vi "Bool Array To Grid.vi"(8 "error in (no error)":errorcluster, 10 "Bool Array In":bool[](array[boolean]), 11 "ElectrodeGrid in":refnum<class "ElectrodeGrid.lvclass">) -> (0 "error out":errorcluster, 2 "Elec Grid Output":bool[][](array[boolean]), 3 "ElectrodeGrid out":refnum<class "ElectrodeGrid.lvclass">)   [LabVIEW 2017, in "ElectrodeGrid.lvclass"]
uses:
  ElectrodeGrid.lvclass
  ElectrodeGrid.lvclass/ElectrodeGrid.ctl
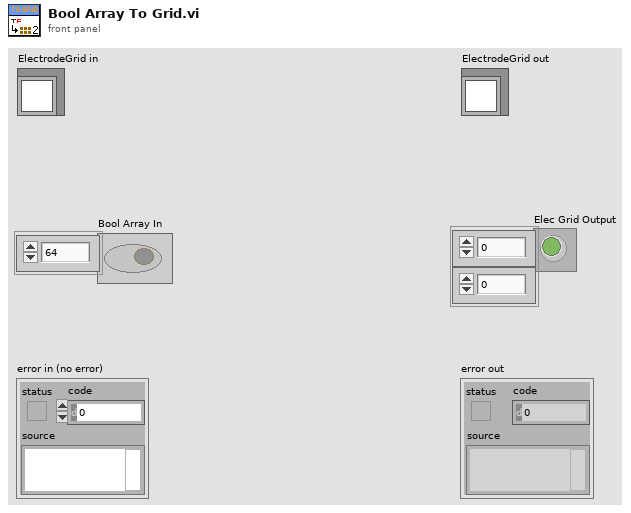
[diagram p1: front panel]
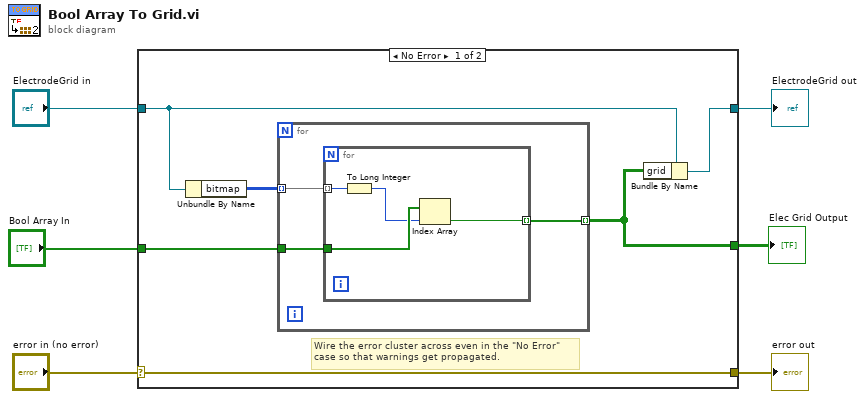
[diagram p0: block diagram]
diagram:
  n1 = case shown="No Error" "error in (no error)" {
    selector: "error in (no error)" -> [w12 w21]
    tunnel: [w12 w21] -> w5
    tunnel: [w7 w20] -> w3
    tunnel: "ElectrodeGrid in" -> [w9 w20]
    tunnel: "Bool Array In" -> [w11 _]
    tunnel: [w8 _] -> w1
    frame No Error {
      # "Wire the error cluster across even in the \"No Error\"\ncase so that warnings get propagated."
      n2 = Unbundle By Name(w9) -> ("bitmap"=w10:u8[][])
      n3 = for {
        tunnel: w11 -> [w15]
        tunnel: w10 -> [w14] mode=indexing
        tunnel: [w13] -> w8 mode=indexing
        n4 = for {
          tunnel: w15 -> [w19]
          tunnel: w14 -> [w18] mode=indexing
          tunnel: [w16] -> w13 mode=indexing
          n5 = To Long Integer(number=w18) -> (32bit integer=w17:i32)
          n6 = Index Array(array=w19, index=w17) -> (element=w16:bool)
        }
      }
      n7 = Bundle By Name(cluster=w9, "grid"=w8) -> (w7:refnum<class "ElectrodeGrid.lvclass">)
    }
    frame Error {
    }
  }
  "error out" <- w5
  "ElectrodeGrid out" <- w3
  "Elec Grid Output" <- w1
